vi "OPERACIONES (SubVI).vi"(1 "Operando 1":dbl, 2 "Enum":T1, 3 "Operando 2":dbl) -> (0 "Salida":dbl)   [LabVIEW 2019]
uses:
  Control 11.ctl
  <vilib>/gmath/NI_Gmath.lvlib
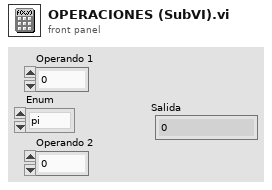
[diagram p1: front panel]
types:
  T1 = typedef "Control 11.ctl" = enum16{"pi", "Tan^(-1)", "Cos^(-1)", "Sin^(-1)", "Tanh", "Cosh", "Sinh", "Tan", "Cos", "Sin", "x^-1", "x!", "e^x", "Log10", "x^1/k", "x^1/3", "x^1/2", "x^3", "x^2", "Log_x", "x^y", "e", "ln", "/", "x", "+", "-"}
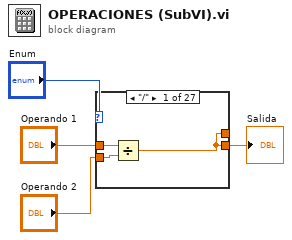
[diagram p0: block diagram]
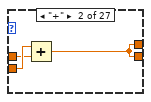
[diagram p2: hidden frame]
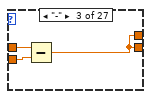
[diagram p3: hidden frame]
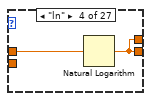
[diagram p4: hidden frame]
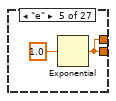
[diagram p5: hidden frame]
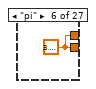
[diagram p6: hidden frame]
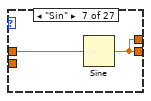
[diagram p7: hidden frame]
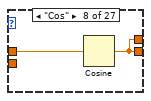
[diagram p8: hidden frame]
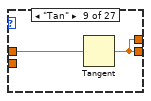
[diagram p9: hidden frame]
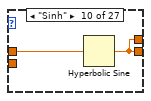
[diagram p10: hidden frame]
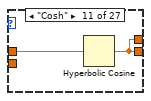
[diagram p11: hidden frame]
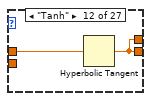
[diagram p12: hidden frame]
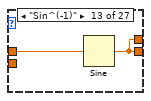
[diagram p13: hidden frame]
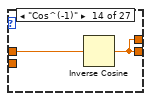
[diagram p14: hidden frame]
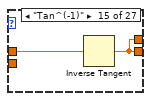
[diagram p15: hidden frame]
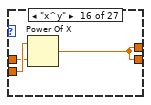
[diagram p16: hidden frame]
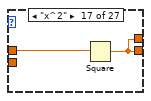
[diagram p17: hidden frame]
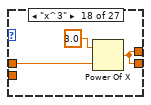
[diagram p18: hidden frame]
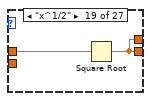
[diagram p19: hidden frame]
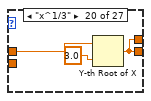
[diagram p20: hidden frame]
diagram:
  n1 = case shown="\"/\"" "Enum" {
    tunnel: "Operando 2" -> [w5 w10 w12 _ _ _ _ _ _ _ _ _ _ _ _ w39 _ _ _ _ w50 w55 w56 _ _ _ _]
    tunnel: "Operando 1" -> [w6 w9 w11 w14 _ _ w19 w21 w23 w25 w27 w29 w31 w33 w35 w37 w40 w42 w45 w47 w51 w54 w57 w59 w61 w63 w65]
    tunnel: [w7 w8 w13 w15 w17 w18 w20 w22 w24 w26 w28 w30 w32 w34 w36 w38 w41 w44 w46 w48 w52 w53 w58 w60 w62 w64 w67] -> w4
    tunnel: [w7 w8 w13 w15 w17 w18 w20 w22 w24 w26 w28 w30 w32 w34 w36 w38 w41 w44 w46 w48 w52 w53 w58 w60 w62 w64 w67] -> _
    frame "/" {
      n2 = Divide(x=w6, y=w5) -> (x/y=w7:dbl)
    }
    frame "+" {
      n3 = Add(x=w10, y=w9) -> (x+y=w8:dbl)
    }
    frame "-" {
      n4 = Subtract(x=w11, y=w12) -> (x-y=w13:dbl)
    }
    frame "ln" {
      n5 = Natural Logarithm(1:w14) -> (0:w15:dbl)
    }
    frame "e" {
      n6 = Exponential(1:1.0 ("x")) -> (0:w17:dbl)
    }
    frame "pi" {
      w18 = 3.141592653589793
    }
    frame "Sin" {
      n7 = Sine(x=w19) -> (sin(x)=w20:dbl)
    }
    frame "Cos" {
      n8 = Cosine(x=w21) -> (cos(x)=w22:dbl)
    }
    frame "Tan" {
      n9 = Tangent(1:w23) -> (0:w24:dbl)
    }
    frame "Sinh" {
      n10 = Hyperbolic Sine(1:w25) -> (0:w26:dbl)
    }
    frame "Cosh" {
      n11 = Hyperbolic Cosine(1:w27) -> (0:w28:dbl)
    }
    frame "Tanh" {
      n12 = Hyperbolic Tangent(1:w29) -> (0:w30:dbl)
    }
    frame "Sin^(-1)" {
      n13 = Sine(x=w31) -> (sin(x)=w32:dbl)
    }
    frame "Cos^(-1)" {
      n14 = Inverse Cosine(1:w33) -> (0:w34:dbl)
    }
    frame "Tan^(-1)" {
      n15 = Inverse Tangent(1:w35) -> (0:w36:dbl)
    }
    frame "x^y" {
      n16 = Power Of X(1:w37, 2:w39) -> (0:w38:dbl)
    }
    frame "x^2" {
      n17 = Square(x=w40) -> (x^2=w41:dbl)
    }
    frame "x^3" {
      n18 = Power Of X(1:w42, 2:3.0 ("x")) -> (0:w44:dbl)
    }
    frame "x^1/2" {
      n19 = Square Root(x=w45) -> (sqrt(x)=w46:dbl)
    }
    frame "x^1/3" {
      n20 = Y-th Root of X(1:3.0 ("x"), 2:w47) -> (0:w48:dbl)
    }
    frame "x^1/k" {
      n21 = Y-th Root of X(1:w50, 2:w51) -> (0:w52:dbl)
    }
    frame "x" {
      n22 = Multiply(x=w55, y=w54) -> (x*y=w53:dbl)
    }
    frame "Log_x" {
      n23 = Logarithm Base X(1:w56, 2:w57) -> (0:w58:dbl)
    }
    frame "Log10" {
      n24 = Logarithm Base 10(1:w59) -> (0:w60:dbl)
    }
    frame "e^x" {
      n25 = Exponential(1:w61) -> (0:w62:dbl)
    }
    frame "x!" {
      n26 = call <vilib>:"Factorial.vi"("n"=w63) -> ("n!"=w64:dbl)  [unwired: 2 in]
    }
    frame "x^-1" {
      n27 = Power Of X(1:w65, 2:-1.0 ("x")) -> (0:w67:dbl)
    }
  }
  "Salida" <- w4
